vi "Module Loop.vi"(8 "error in (no error)":errorcluster, 11 "Data Logger Module in":refnum<class "Data Logger DBL Module.lvclass">) -> (0 "error out":errorcluster, 3 "Data Logger Module out":refnum<class "Data Logger DBL Module.lvclass">)   [LabVIEW 2020, in "VolatusData.lvlib" / "Data Logger DBL Module.lvclass"]
uses:
  Data Logger DBL Module.lvclass
  C:/dev/lv20CE/relink/lv-volatus/Volatus/Module/Module.lvclass
  Data Logger DBL Module.lvclass/Data Logger DBL Module.ctl
  Volatus/Module/Module.lvclass
  New Data.ctl
  Prepare Log.ctl
  Logger State.ctl
  Logger Started.ctl
  Volatus/Module/Module.lvclass/Module.ctl
  Volatus/MessageQ/MessageQ.lvclass/MessageQ.ctl
  Volatus/Module/Parent Q.vi
  Volatus/Module/Update Substatus.vi
  <vilib>/Utility/error.llb/Error Cluster From Error Code.vi
  VolatusData.lvlib
  Volatus/MessageQ/MessageQ.lvclass
  lv-promises/Promises/Promise/Promise.lvclass
panel:
  out "Parent Name":string
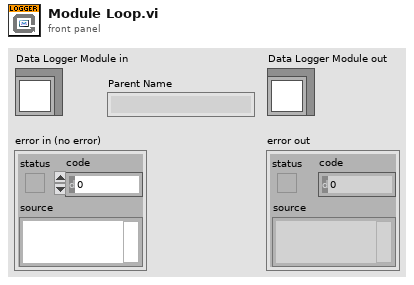
[diagram p1: front panel]
types:
  T1 = enum32{"Invalid", "Standard", "Closed", "Hidden", "Minimized", "Maximized"}
  T2 = typedef "VolatusData.lvlib/New Data.ctl" = cluster{"Channels":waveform(dbl)[]}
  T3 = typedef "VolatusData.lvlib/Prepare Log.ctl" = cluster{"Folder":path, "Series":string}
  T4 = typedef "VolatusData.lvlib/Logger State.ctl" = enum16{"Unknown", "Idle", "Preparing", "Ready", "Logging", "Stopping"}
  T5 = typedef "VolatusData.lvlib/Logger Started.ctl" = cluster{"ID":string}
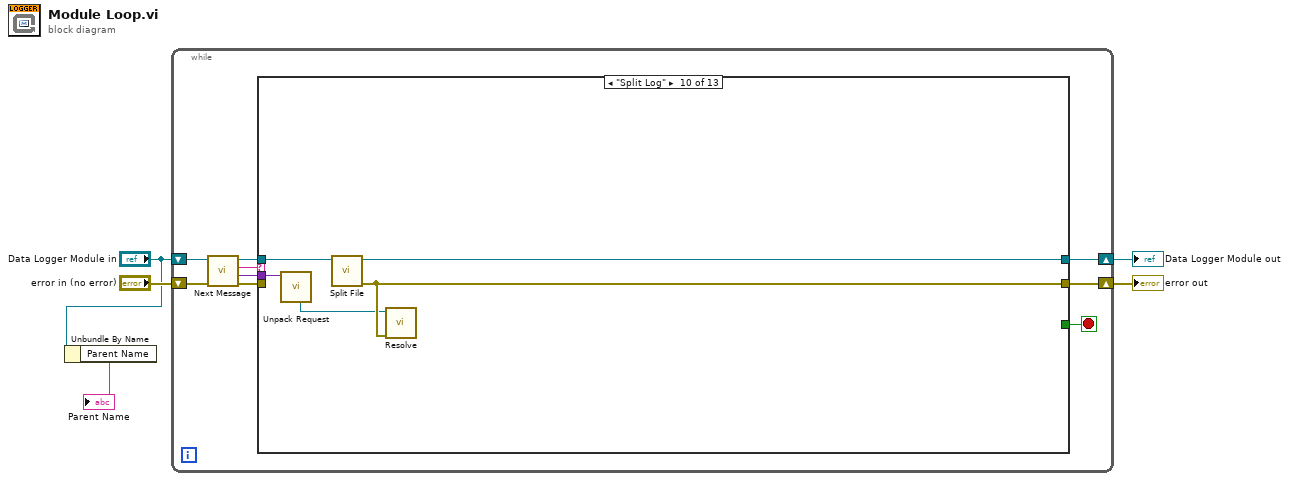
[diagram p0: block diagram]
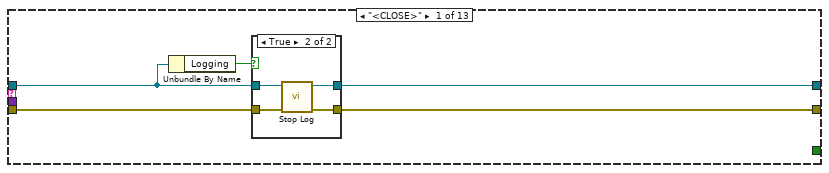
[diagram p2: hidden frame]
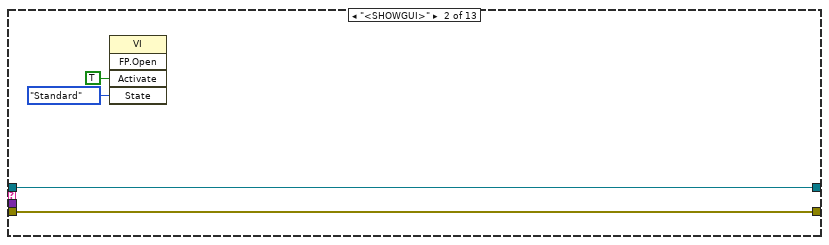
[diagram p4: hidden frame]
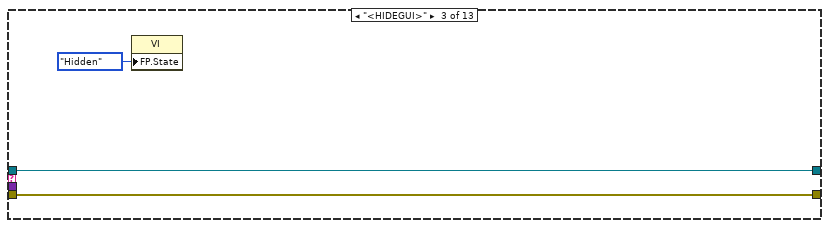
[diagram p5: hidden frame]
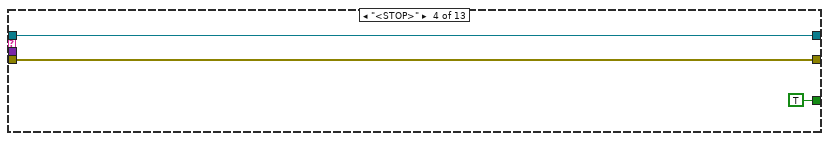
[diagram p6: hidden frame]
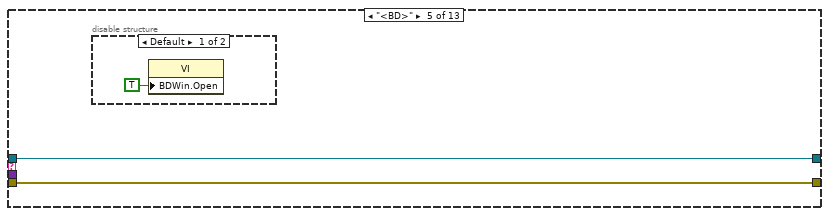
[diagram p7: hidden frame]
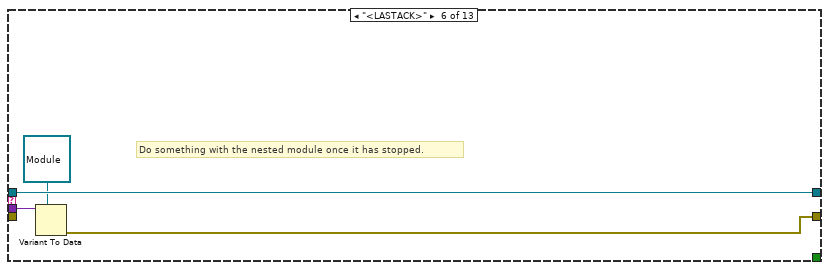
[diagram p9: hidden frame]
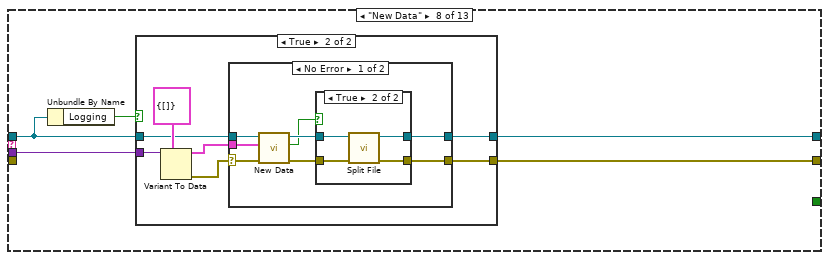
[diagram p11: hidden frame]
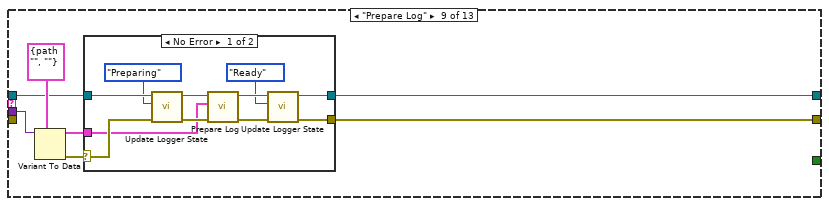
[diagram p15: hidden frame]
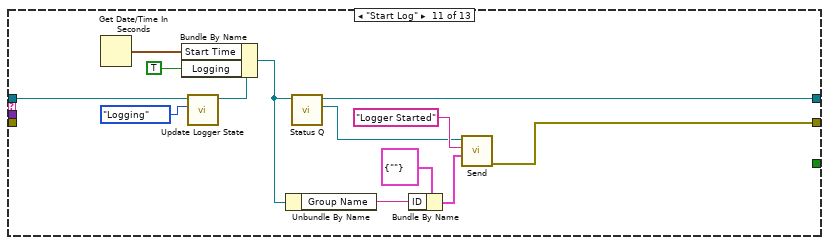
[diagram p17: hidden frame]
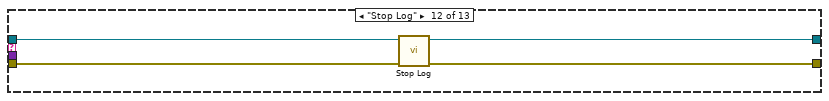
[diagram p18: hidden frame]
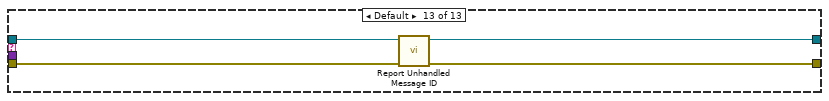
[diagram p19: hidden frame]
diagram:
  n1 = Unbundle By Name("Data Logger Module in") -> ("Parent Name"=→"Parent Name":string)
  n2 = while {
    shift-right: [w9] -> w4
    shift-left: "Data Logger Module in" -> [w14]
    shift-right: [w8] -> w3
    shift-left: "error in (no error)" -> [w13]
    stop <- w7 stop-if-true
    n3 = call "Next Message.vi"("error in (no error)"=w13, "Module in"=w14) -> ("error out"=w12:errorcluster, "Data"=w6:variant, "ID"=w11:string, "Module out"=w10:refnum<class "Data Logger DBL Module.lvclass">)  [unwired: 6 in]
    n4 = case shown="\"Split Log\"" w11 {
      tunnel: w12 -> [w19 w28 w31 w34 w36 _ w43 _ _ _ _ w115 w119]
      tunnel: w10 -> [w16 w29 w32 w35 w37 w42 w44 w47 w76 w97 w106 w113 w117]
      tunnel: [w17 w29 w32 w35 w37 w42 w44 w46 w75 w96 w103 w112 w116] -> w9
      tunnel: [w18 w28 w31 w34 w36 w39 w43 w45 w74 w98 w107 w114 w118] -> w8
      tunnel: [_ _ _ TRUE _ _ _ _ _ _ _ _ _] -> w7
      tunnel: w6 -> [_ _ _ _ _ w41 _ w49 w80 w95 _ _ _]
      frame "<CLOSE>" {
        n5 = Unbundle By Name(w16) -> ("Logging"=w15:bool)
        n6 = case shown="True" w15 {
          tunnel: w19 -> [w20 w25]
          tunnel: [w20 w24] -> w18
          tunnel: [w21 w23] -> w17
          tunnel: w16 -> [w21 w22]
          frame False {
          }
          frame True {
            n7 = call "Stop Log.vi"("error in (no error)"=w25, "Data Logger Module in"=w22) -> ("error out"=w24:errorcluster, "Data Logger Module out"=w23:refnum<class "Data Logger DBL Module.lvclass">)  [unwired: 8 in]
          }
        }
      }
      frame "<SHOWGUI>" {
        n8 = invoke class="VI" method="FP.Open"("Activate"=TRUE ("Activate?"), "State"=T1."Standard") -> ()  [unwired: 3 in, 5 out]
      }
      frame "<HIDEGUI>" {
        n9 = property class="VI"("FP.State"=T1."Hidden" ("Front Panel Window:State")) -> ()  [unwired: 2 in, 2 out]
      }
      frame "<STOP>" {
      }
      frame "<BD>" {
        n10 = disable-structure shown="Default" {
          frame condition #0 (active) {
            n11 = property class="VI"("BDWin.Open"=TRUE ("Block Diagram Window:Open")) -> ()  [unwired: 2 in, 2 out]
          }
          frame condition #1 {
          }
        }
      }
      frame "<LASTACK>" {
        # "Do something with the nested module once it has stopped."
        n12 = Variant To Data(type=refnum<class "Module.lvclass"> refnum ("Volatus:Module"), Variant=w41) -> (error out=w39:errorcluster)  [unwired: 1 in, 1 out]
      }
      frame "<TIMEOUT>" {
        # "No message for this module was received in time"
      }
      frame "New Data" {
        n13 = Unbundle By Name(w47) -> ("Logging"=w48:bool)
        n14 = case shown="True" w48 {
          tunnel: w49 -> [_ w57]
          tunnel: w47 -> [w50 w55]
          tunnel: [w50 w52] -> w46
          tunnel: [_ w51] -> w45
          frame False {
          }
          frame True {
            n15 = Variant To Data(type=T2 {"Channels"=[]} ("New Data"), Variant=w57) -> (data=w54:T2, error out=w53:errorcluster)  [unwired: 1 in]
            n16 = case shown="No Error" w53 {
              selector: w53 -> [w63 w73]
              tunnel: w55 -> [w65 w72]
              tunnel: w54 -> [w64 _]
              tunnel: [w59 w72] -> w52
              tunnel: [w61 w73] -> w51
              frame No Error {
                n17 = call "New Data.vi"("error in (no error)"=w63, "New Data"=w64, "Data Logger Module in"=w65) -> ("error out"=w62:errorcluster, "Split"=w58:bool, "Data Logger Module out"=w60:refnum<class "Data Logger DBL Module.lvclass">)  [unwired: 6 in]
                n18 = case shown="True" w58 {
                  tunnel: w62 -> [w66 w71]
                  tunnel: [w66 w70] -> w61
                  tunnel: w60 -> [w67 w69]
                  tunnel: [w67 w68] -> w59
                  frame False {
                  }
                  frame True {
                    n19 = call "Split File.vi"("error in (no error)"=w71, "Data Logger Module in"=w69) -> ("error out"=w70:errorcluster, "Data Logger Module out"=w68:refnum<class "Data Logger DBL Module.lvclass">)  [unwired: 8 in]
                  }
                }
              }
              frame Error {
              }
            }
          }
        }
      }
      frame "Prepare Log" {
        n20 = Variant To Data(type=T3 {"Folder"=path "", "Series"=""} ("Prepare Log"), Variant=w80) -> (data=w77:T3, error out=w78:errorcluster)  [unwired: 1 in]
        n21 = case shown="No Error" w78 {
          selector: w78 -> [w90 w92]
          tunnel: w77 -> [w89 _]
          tunnel: w76 -> [w83 w93]
          tunnel: [w85 w93] -> w75
          tunnel: [w87 w92] -> w74
          frame No Error {
            n22 = call "Update Logger State.vi"("error in (no error)"=w90, "Logger State"=Logger_State."Preparing", "Module in"=w83) -> ("error out"=w91:errorcluster, "Module"=w82:refnum<class "Data Logger DBL Module.lvclass">)  [unwired: 7 in]
            n23 = call "Prepare Log.vi"("error in (no error)"=w91, "Prepare Log"=w89, "Data Logger Module in"=w82) -> ("error out"=w88:errorcluster, "Data Logger Module out"=w86:refnum<class "Data Logger DBL Module.lvclass">)  [unwired: 7 in]
            n24 = call "Update Logger State.vi"("error in (no error)"=w88, "Logger State"=Logger_State."Ready", "Module in"=w86) -> ("error out"=w87:errorcluster, "Module"=w85:refnum<class "Data Logger DBL Module.lvclass">)  [unwired: 7 in]
          }
          frame Error {
          }
        }
      }
      frame "Split Log" {
        n25 = call "Unpack Request.vi"("Request Data"=w95) -> ("Promise"=w94:refnum<class "Promise.lvclass">)  [unwired: 8 in, 2 out]
        n26 = call "Split File.vi"("Data Logger Module in"=w97) -> ("error out"=w98:errorcluster, "Data Logger Module out"=w96:refnum<class "Data Logger DBL Module.lvclass">)  [unwired: 9 in]
        n27 = call "Resolve.vi"("error in (no error)"=w98, "Promise in"=w94) -> ()  [unwired: 8 in, 2 out]
      }
      frame "Start Log" {
        n28 = Get Date/Time In Seconds() -> (seconds since 1Jan1904=w99:timestamp)
        n29 = call "Update Logger State.vi"("Logger State"=Logger_State."Logging", "Module in"=w106) -> ("Module"=w105:refnum<class "Data Logger DBL Module.lvclass">)  [unwired: 8 in, 1 out]
        n30 = Bundle By Name(cluster=w105, "Start Time"=w99, "Logging"=TRUE) -> (w101:refnum<class "Data Logger DBL Module.lvclass">)
        n31 = Unbundle By Name(w101) -> ("Group Name"=w100:string)
        n32 = call "Status Q.vi"("Data Logger Module in"=w101) -> ("Status Q"=w102:refnum<class "MessageQ.lvclass">, "Data Logger Module out"=w103:refnum<class "Data Logger DBL Module.lvclass">)  [unwired: 9 in]
        n33 = Bundle By Name(cluster=T5 {"ID"=""} ("Logger Started"), "ID"=w100) -> (w109:T5)
        n34 = call "Send.vi"("Data"=w109, "ID"="Logger Started", "MessageQ in"=w102) -> ("error out"=w107:errorcluster)  [unwired: 7 in, 1 out]
      }
      frame "Stop Log" {
        n35 = call "Stop Log.vi"("error in (no error)"=w115, "Data Logger Module in"=w113) -> ("error out"=w114:errorcluster, "Data Logger Module out"=w112:refnum<class "Data Logger DBL Module.lvclass">)  [unwired: 8 in]
      }
      frame Default {
        n36 = call "Report Unhandled Message ID.vi"("error in (no error)"=w119, "Module in"=w117) -> ("error out"=w118:errorcluster, "Module out"=w116:refnum<class "Data Logger DBL Module.lvclass">)  [unwired: 8 in]
      }
    }
  }
  "error out" <- w3
  "Data Logger Module out" <- w4
